vi "test Correct Amount of Labels In Log.vi"(8 "error in (no error)":errorcluster, 11 "TestCase in":refnum<class "Acyclic Logging Loopback.lvclass">) -> (0 "error out":errorcluster, 3 "TestCase out":refnum<class "Acyclic Logging Loopback.lvclass">)   [LabVIEW 2020, in "Acyclic Logging Loopback.lvclass"]
uses:
  Acyclic Logging Loopback.lvclass
  Acyclic Logging Loopback.lvclass/Acyclic Logging Loopback.ctl
  <vilib>/addons/_JKI Toolkits/VI Tester/TestCase.llb/TestCase.lvclass
  <vilib>/NI VeriStand/Execution/Workspace/NI_VS Workspace ExecutionAPI.lvlib
  <vilib>/NI VeriStand/Execution/Workspace/NI VeriStand - Set Multiple Channel Values.vi
  niveristand-custom-device-testing-tools/VeriStandTestUtilities/VeriStandTestUtilities.lvlib
  <vilib>/WebDAVClient/NI_WebDAV.lvlib
  <vilib>/WebDAVClient/Advanced/Get Buffer.vi
  C:/dev/git/niveristand-custom-device-testing-tools/VeriStandTestCase/VeriStandTestCase.lvclass
  C:/Program Files (x86)/National Instruments/LabVIEW 2020/vi.lib/addons/_JKI Toolkits/VI Tester/TestCase.llb/TestCase.lvclass
  C:/dev/git/niveristand-ballard-arinc429-custom-device/Source/Custom Device Support/Tests/System/Acyclic Logging Loopback/Acyclic Logging Loopback.lvclass
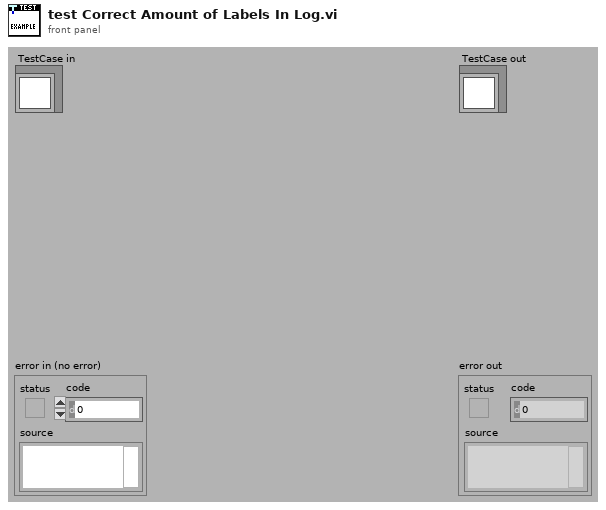
[diagram p1: front panel]
types:
  T1 = typedef "NI_WebDAV.lvlib/SessionHandle.ctl" = refnum<k1>
  T2 = typedef "NI_VS Workspace ExecutionAPI.lvlib/WorkspaceAPI.ctl" = refnum<k24>
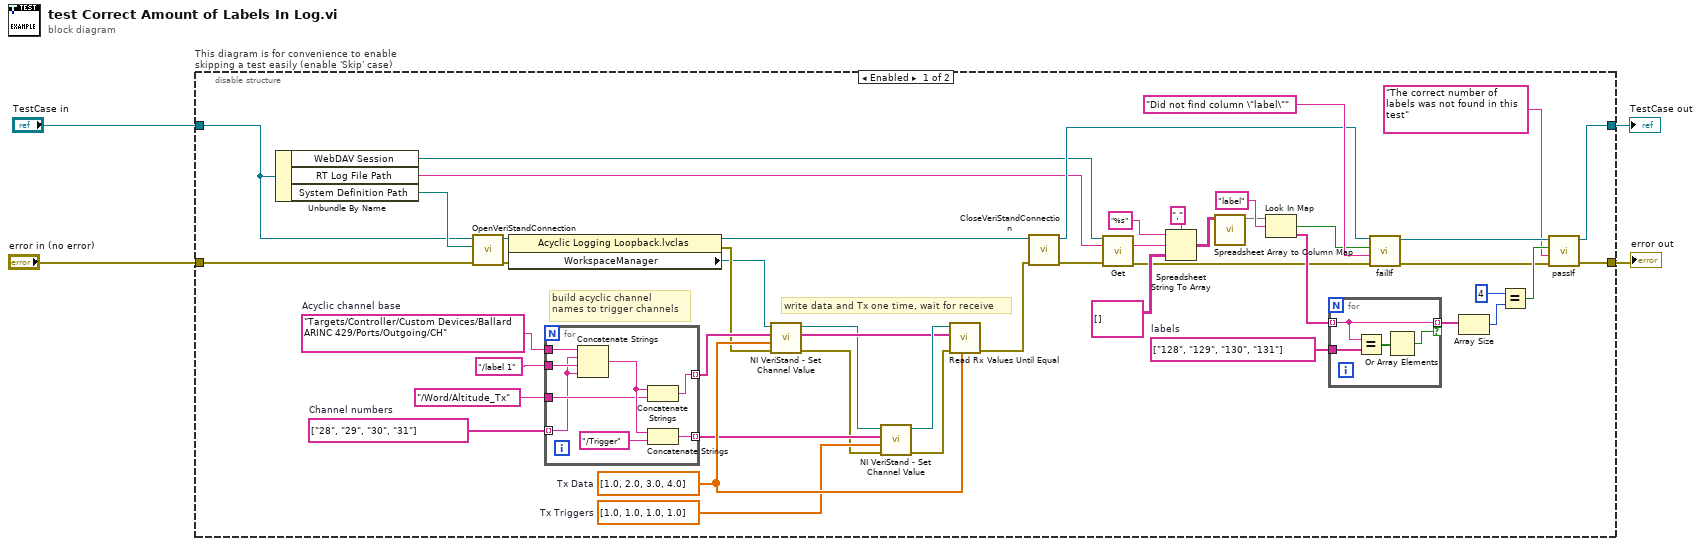
[diagram p0: block diagram]
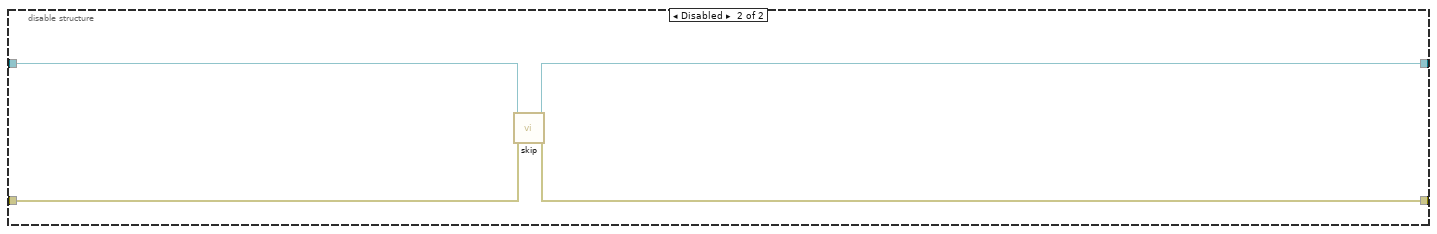
[diagram p2: hidden frame]
diagram:
  n1 = disable-structure "This diagram is for convenience to enable skipping a test easily (enable 'Skip' case)" shown="Enabled" {
    disable-tunnel: "TestCase in" -> [w10 w66]
    disable-tunnel: [w6 w64] -> w1
    disable-tunnel: [w5 w65] -> w3
    disable-tunnel: "error in (no error)" -> [w9 w63]
    frame Enabled {
      w46 = string[] ["128", "129", "130", "131"]  # labels
      w38 = dbl[] [1.0, 1.0, 1.0, 1.0]  # Tx Triggers
      w42 = dbl[] [1.0, 2.0, 3.0, 4.0]  # Tx Data
      w29 = string[] ["28", "29", "30", "31"]  # Channel numbers
      w28 = "Targets/Controller/Custom Devices/Ballard ARINC 429/Ports/Outgoing/CH"  # Acyclic channel base
      # "write data and Tx one time, wait for receive"
      # "build acyclic channel\nnames to trigger channels"
      n2 = Unbundle By Name(w10) -> ("WebDAV Session"=w15:T1, "RT Log File Path"=w16:string, "System Definition Path"=w12:path)
      n3 = call-dynamic "OpenVeriStandConnection.vi"("error in (no error)"=w9, "System Definition File"=w12, "VeriStand Test Case in"=w10) -> ("error out"=w11:errorcluster, "VeriStand Test Case out"=w31:refnum<class "Acyclic Logging Loopback.lvclass">)  [unwired: 6 in, 1 out]
      n4 = property class="Acyclic Logging Loopback.lvclas"(reference=w31, error in=w11) -> (reference out=w32:refnum<class "Acyclic Logging Loopback.lvclass">, error out=w34:errorcluster, "WorkspaceManager"=w33:T2)
      n5 = for {
        tunnel: w28 -> [w62]
        tunnel: w29 -> [w55] mode=indexing
        tunnel: "/label 1" -> [w61]
        tunnel: [w58] -> w39 mode=indexing
        tunnel: [w59] -> w37 mode=indexing
        tunnel: "/Word/Altitude_Tx" -> [w56]
        n6 = Concatenate Strings(w62, w55, w61, w55) -> (w57:string)
        n7 = Concatenate Strings(w57, w56) -> (w58:string)
        n8 = Concatenate Strings(w57, "/Trigger") -> (w59:string)
      }
      n9 = call-poly <vilib>:"NI VeriStand - Set Channel Value.vi"("error in (no error)"=w34, "Values"=w42, "Channels"=w39, "WorkspaceManager in"=w33) -> ("error out"=w36:errorcluster, "WorkspaceManager out"=w35:T2)  [unwired: 6 in]
      n10 = call-poly <vilib>:"NI VeriStand - Set Channel Value.vi"("error in (no error)"=w36, "Values"=w38, "Channels"=w37, "WorkspaceManager in"=w35) -> ("error out"=w40:errorcluster, "WorkspaceManager out"=w41:T2)  [unwired: 6 in]
      n11 = call "Read Rx Values Until Equal.vi"("expected values"=w42, "error in"=w40, "Rx aliases"=w39, "workspace manager in"=w41) -> ("error out"=w43:errorcluster)  [unwired: 5 in, 2 out]
      n12 = call-dynamic "CloseVeriStandConnection.vi"("error in (no error)"=w43, "VeriStand Test Case in"=w32) -> ("error out"=w13:errorcluster, "VeriStand Test Case out"=w24:refnum<class "Acyclic Logging Loopback.lvclass">)  [unwired: 8 in]
      n13 = call-poly <vilib>:"Get.vi"("session handle"=w15, "relative uri"=w16, "error in (no error)"=w13) -> ("data"=w17:string, "error out"=w14:errorcluster)  [unwired: 10 in, 1 out]
      n14 = Spreadsheet String To Array(delimiter (Tab)=",", format string="%s", spreadsheet string=w17, array type (2D Dbl)=string[][] []) -> (array=w8:string[][])
      n15 = call "Spreadsheet Array to Column Map.vi"("array"=w8) -> ("map"=w7:map{string, string[]})  [unwired: 10 in]
      n16 = Look In Map(map=w7, key="label") -> (key not found?=w26:bool, value=w45:string[])  [unwired: 1 in]
      n17 = for {
        tunnel: w45 -> [w52] mode=indexing
        tunnel: w46 -> [w54]
        tunnel: [w52] -> w47 mode=indexing if=w51
        n18 = Equal?(x=w52, y=w54) -> (x = y?=w53:bool[])
        n19 = Or Array Elements(Boolean array=w53) -> (logical OR=w51:bool)
      }
      n20 = call-dynamic "failIf.vi"("error in (no error)"=w14, "message (\"\")"="Did not find column \"label\"" ("message (\"\")"), "fail"=w26, "TestCase in"=w24) -> ("error out"=w23:errorcluster, "TestCase out"=w25:refnum<class "Acyclic Logging Loopback.lvclass">)  [unwired: 6 in]
      n21 = Array Size(array=w47) -> (size(s)=w48:i32)
      n22 = Equal?(x=4, y=w48) -> (x = y?=w50:bool)
      n23 = call-dynamic "passIf.vi"("error in (no error)"=w23, "message (\"\")"="The correct number of labels was not found in this test" ("message (\"\")"), "pass"=w50, "TestCase in"=w25) -> ("error out"=w5:errorcluster, "TestCase out"=w6:refnum<class "Acyclic Logging Loopback.lvclass">)  [unwired: 6 in]
    }
    frame Disabled {
      # "skip test result while test is under development"
      n24 = call <vilib>:"skip.vi"("error in (no error)"=w63, "TestCase in"=w66) -> ("error out"=w65:errorcluster, "TestCase out"=w64:refnum<class "Acyclic Logging Loopback.lvclass">)  [unwired: 8 in]
    }
  }
  "error out" <- w3
  "TestCase out" <- w1
